vi "stop.vi"(8 "error in (no error)":errorcluster, 11 "HGF_DSCMonitor in":refnum<class "HGF_DSCMonitor.lvclass">) -> (0 "error out":errorcluster, 3 "HGF_DSCMonitor out":refnum<class "HGF_DSCMonitor.lvclass">)   [LabVIEW 2012, in "HGF_DSC.lvlib" / "HGF_DSCMonitor.lvclass"]
uses:
  HGF_DSCMonitor.lvclass
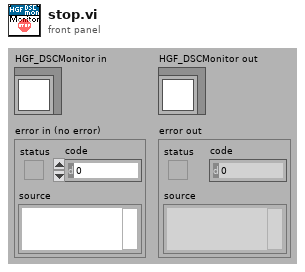
[diagram p1: front panel]
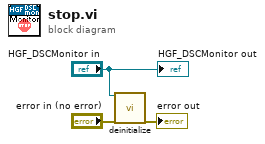
[diagram p0: block diagram]
diagram:
  n1 = call-dynamic "deinitialize.vi"("HGF_DSCMonitor"="HGF_DSCMonitor in", "error in (no error)"="error in (no error)") -> ("error out"=→"error out":errorcluster)  [unwired: 17 in]
  "HGF_DSCMonitor out" <- "HGF_DSCMonitor in"
